vi "LEP_RV_GetTCPDebugHostIP.vi"() -> (0 "IP Address":string)   [LabVIEW 2011]
uses:
  <vilib>/Platform/EmbProject/Plugins/utilities/LEP_Utilities_GetSetProjectData_String.vi
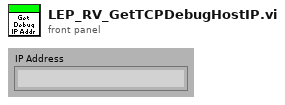
[diagram p1: front panel]
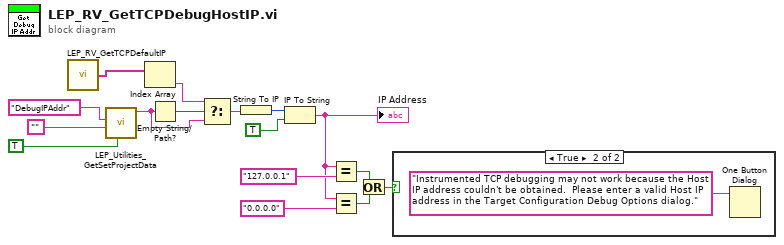
[diagram p0: block diagram]
diagram:
  n1 = call "LEP_RV_GetTCPDefaultIP.vi"() -> ("IP address"=w2:string[])  [unwired: 1 in]
  n2 = call-poly <vilib>:"LEP_Utilities_GetSetProjectData.vi"("access target data (F)"=TRUE, "data in"="", "ItemName"="DebugIPAddr") -> ("data out"=w12:string)  [unwired: 6 in, 2 out]
  n3 = Index Array(array=w2) -> (element=w1:string)  [unwired: 1 in]
  n4 = Empty String/Path?(string/path=w12) -> (empty?=w13:bool)
  n5 = Select(t=w1, s=w13, f=w12) -> (s? t:f=w8:string)
  n6 = String To IP(1:w8) -> (0:w10:u32)
  n7 = IP To String(1:TRUE ("dot notation? (F)"), 2:w10) -> (0:w6:string)
  "IP Address" <- w6
  n8 = Equal?(x=w6, y="127.0.0.1") -> (x = y?=w5:bool)
  n9 = Equal?(x=w6, y="0.0.0.0") -> (x = y?=w4:bool)
  n10 = Or(x=w5, y=w4) -> (x .or. y?=w3:bool)
  n11 = case shown="True" w3 {
    frame False {
    }
    frame True {
      n12 = One Button Dialog(message="Instrumented TCP debugging may not work because the Host IP address couldn't be obtained.  Please enter a valid Host IP address in the Target Configuration Debug Options dialog.") -> ()  [unwired: 1 in, 1 out]
    }
  }
